vi "SingleOutput_GSM-20H10.vi"(0 "VISA resource name":refnum<visa-resource-name>="USB0::0x2184::0x007D::gew872418::INSTR", 1 "Source Mode  (0: Voltage)":u16(ring) items=["Voltage", "Current"], 2 "Output Level (0)":dbl=1.7, 3 "Compliance  Level (0.1)":dbl=0.001, 4 "stop":bool) -> (6 "Voltage":sgl=1.699984, 7 "Current":sgl=0.000169597, 8 "Resistance":sgl=10023.67)   [LabVIEW 2016]
uses:
  <instrlib>/GSM Series/GSM.lvlib
panel:
  out "IV":cluster{dbl[], dbl[]}(graph)
  in  "Enable Resistance Auto Range (T:Enable)":bool=TRUE
  in  "Enable Current Auto Range (T:Enable)":bool=TRUE
  in  "Enable Voltage Auto Range (T:Enable)":bool=TRUE
  in  "Resistance Manual Range (1.0)":dbl=1.0
  in  "Current Manual Range (1.0)":dbl=1.0
  in  "Voltage Manual Range (1.0)":dbl=1.0
  in  "Serial Configuration":T1={"Baud Rate"=9600, "Parity"=0, "Data Bits"=8, "Stop Bits"=10, "Flow Control"=0} {"Flow Control" items=["None", "XON/XOFF", "RTS/CTS", "XON/XOFF & RTS/CTS", "DTR/DSR", "XON/XOFF & DTR/DSR"]; "Stop Bits" items=["1.0"=10, "1.5"=15, "2.0"=20]; "Data Bits" items=["7"=7, "8"=8]; "Parity" items=["None", "Odd", "Even", "Mark", "Space"]; "Baud Rate" items=["300"=300, "600"=600, "1200"=1200, "2400"=2400, "4800"=4800, "9600"=9600, "19200"=19200]}
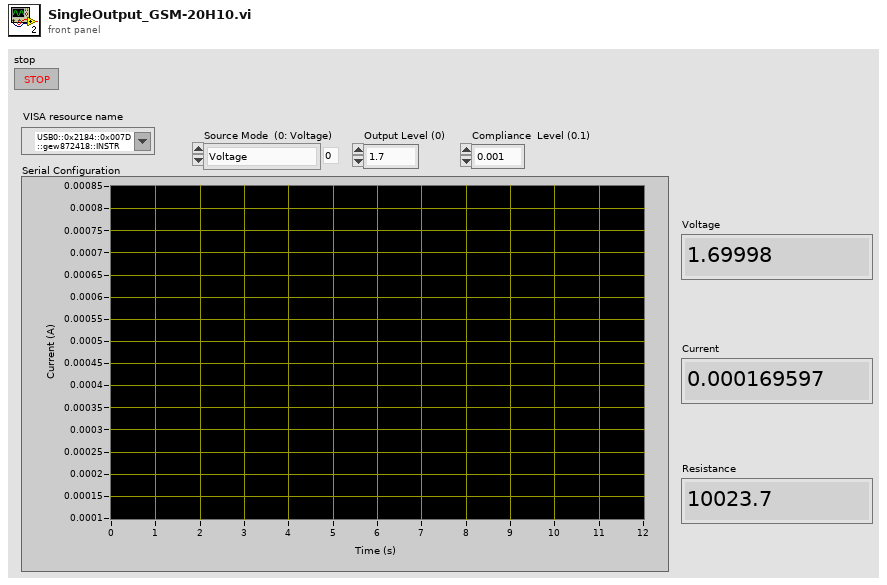
[diagram p1: front panel]
types:
  T1 = cluster{"Baud Rate":u32, "Parity":u16, "Data Bits":u16, "Stop Bits":u16, "Flow Control":u16}
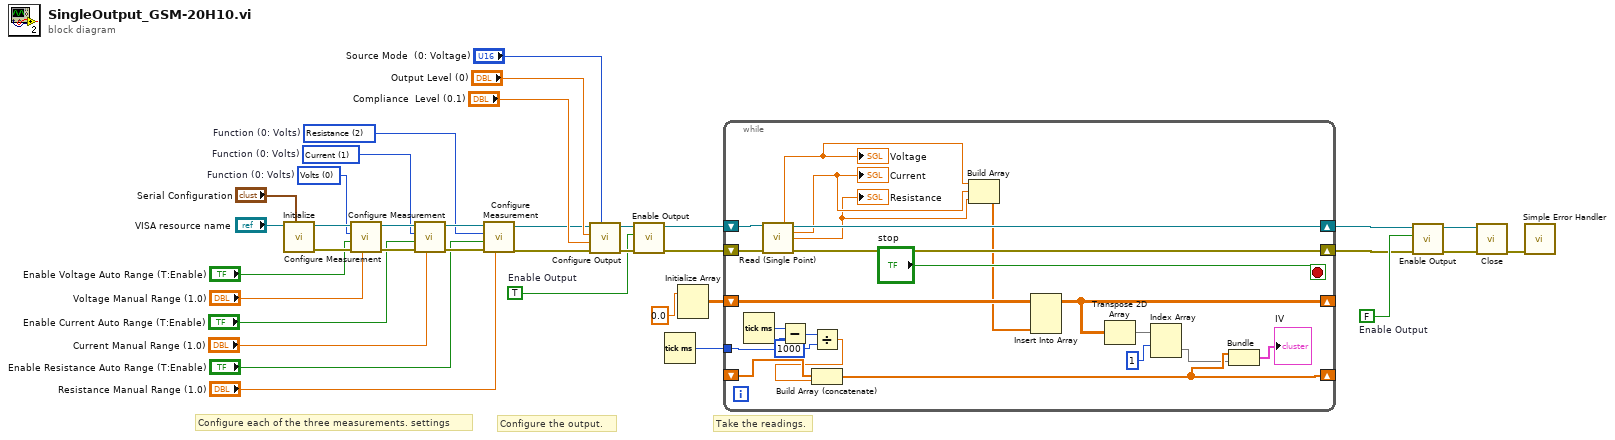
[diagram p0: block diagram]
diagram:
  w7 = TRUE  # Enable Output
  w18 = FALSE  # Enable Output
  w25 = u16 2 items=["Volts", "Current", "Resistance"]  # Function (0: Volts)
  w26 = u16 1 items=["Volts", "Current", "Resistance"]  # Function (0: Volts)
  w27 = u16 0 items=["Volts", "Current", "Resistance"]  # Function (0: Volts)
  # "Take the readings."
  # "Configure the output."
  # "Configure each of the three measurements. settings"
  n1 = call <instrlib>:"Initialize.vi"("Serial Configuration"="Serial Configuration", "VISA resource name"="VISA resource name") -> ("error out"=w32:errorcluster, "VISA resource name out"=w33:refnum<visa-resource-name>)  [unwired: 8 in]
  n2 = call <instrlib>:"Configure Measurement.vi"("Manual Range (1.0)"="Voltage Manual Range (1.0)", "error in (no error)"=w32, "Enable Auto Range (T:Enable)"="Enable Voltage Auto Range (T:Enable)", "Function (0: Volts)"=w27, "VISA resource name"=w33) -> ("error out"=w30:errorcluster, "VISA resource name out"=w31:refnum<visa-resource-name>)  [unwired: 5 in]
  n3 = call <instrlib>:"Configure Measurement.vi"("Manual Range (1.0)"="Current Manual Range (1.0)", "error in (no error)"=w30, "Enable Auto Range (T:Enable)"="Enable Current Auto Range (T:Enable)", "Function (0: Volts)"=w26, "VISA resource name"=w31) -> ("error out"=w29:errorcluster, "VISA resource name out"=w28:refnum<visa-resource-name>)  [unwired: 5 in]
  n4 = call <instrlib>:"Configure Measurement.vi"("Manual Range (1.0)"="Resistance Manual Range (1.0)", "error in (no error)"=w29, "Enable Auto Range (T:Enable)"="Enable Resistance Auto Range (T:Enable)", "Function (0: Volts)"=w25, "VISA resource name"=w28) -> ("error out"=w6:errorcluster, "VISA resource name out"=w5:refnum<visa-resource-name>)  [unwired: 5 in]
  n5 = call <instrlib>:"Configure Output.vi"("Source Mode  (0: Voltage)"="Source Mode  (0: Voltage)", "error in (no error)"=w6, "Compliance  Level (0.1)"="Compliance  Level (0.1)", "Output Level (0)"="Output Level (0)", "VISA resource name"=w5) -> ("error out"=w8:errorcluster, "VISA resource name out"=w9:refnum<visa-resource-name>)  [unwired: 5 in]
  n6 = call <instrlib>:"Enable Output.vi"("error in (no error)"=w8, "Enable Output (T: Enable)"=w7, "VISA resource name"=w9) -> ("error out"=w11:errorcluster, "VISA resource name out"=w10:refnum<visa-resource-name>)  [unwired: 7 in]
  n7 = Tick Count (ms)() -> (millisecond timer value=w1:u32)
  n8 = Initialize Array(0.0 ("element")) -> (w2:dbl[][])  [unwired: 2 in]
  n9 = while {
    shift-right: [w58] -> w13
    shift-left: w11 -> [w56]
    shift-right: [w57] -> w12
    shift-left: w10 -> [w55]
    shift-right: [w48] -> _
    shift-left: w2 -> [w50]
    shift-right: [w43] -> _
    shift-left: _ -> [w45]
    tunnel: w1 -> [w40]
    stop <- "stop" stop-if-true
    n10 = Tick Count (ms)() -> (millisecond timer value=w41:u32)
    n11 = call <instrlib>:"Read (Single Point).vi"("VISA resource name"=w55, "error in (no error)"=w56) -> ("Voltage"=w53:sgl, "VISA resource name out"=w57:refnum<visa-resource-name>, "Current"=w52:sgl, "Resistance"=w51:sgl, "error out"=w58:errorcluster)  [unwired: 7 in, 2 out]
    "Voltage" <- w53
    "Current" <- w52
    "Resistance" <- w51
    n12 = Subtract(x=w41, y=w40) -> (x-y=w39:u32)
    n13 = Divide(x=w39, y=u32 1000) -> (x/y=w37:dbl)
    n14 = Build Array (concatenate)(w45, w37) -> (w43:dbl[])
    n15 = Build Array(w53, w52, w51) -> (w49:sgl[])
    n16 = Insert Into Array(array=w50, new element=w49) -> (w48:dbl[][])  [unwired: 2 in]
    n17 = Transpose 2D Array(2D array=w48) -> (transposed array=w47:dbl[][])
    n18 = Index Array(array=w47, index (row)=1) -> (element=w42:dbl[])  [unwired: 1 in]
    n19 = Bundle(w43, w42) -> (→"IV":cluster{dbl[], dbl[]})  [unwired: 1 in]
  }
  n20 = call <instrlib>:"Enable Output.vi"("error in (no error)"=w13, "Enable Output (T: Enable)"=w18, "VISA resource name"=w12) -> ("error out"=w14:errorcluster, "VISA resource name out"=w15:refnum<visa-resource-name>)  [unwired: 7 in]
  n21 = call <instrlib>:"Close.vi"("error in (no error)"=w14, "VISA resource name"=w15) -> ("error out"=w36:errorcluster)  [unwired: 9 in]
  n22 = call <vilib>:"Simple Error Handler.vi"("error in (no error)"=w36) -> ()  [unwired: 4 in, 5 out]
